vi "Raise Required Override Error.vi"(0 "RFFE Command in":refnum<class "RFFE Command.lvclass">, 5 "VI Refnum in (This VI)":refnum<vi>, 11 "error in (no error)":errorcluster) -> (4 "RFFE Command out":refnum<class "RFFE Command.lvclass">, 6 "VI Refnum out":refnum<vi>, 15 "error out":errorcluster)   [LabVIEW 2018, in "MIPI RFFE API.lvlib" / "RFFE Command.lvclass"]
uses:
  RFFE Command.lvclass
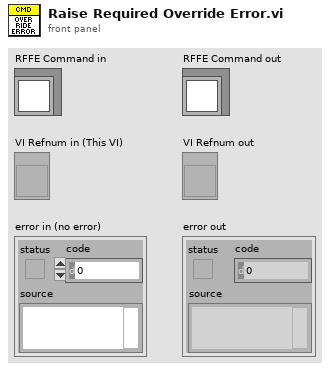
[diagram p1: front panel]
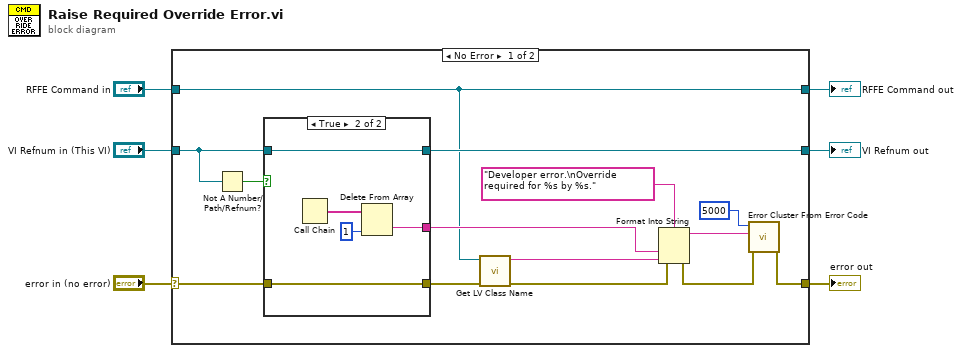
[diagram p0: block diagram]
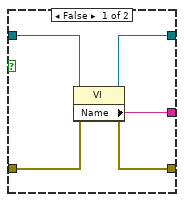
[diagram p2: hidden frame]
diagram:
  n1 = case shown="No Error" "error in (no error)" {
    selector: "error in (no error)" -> [w13 w33]
    tunnel: [w16 w33] -> w5
    tunnel: "VI Refnum in (This VI)" -> [w14 w32]
    tunnel: [w12 w32] -> w3
    tunnel: "RFFE Command in" -> [w7 w31]
    tunnel: [w7 w31] -> w1
    frame No Error {
      n2 = Not A Number/Path/Refnum?(number/path/refnum=w14) -> (NaN/Path/Refnum?=w15:bool)
      n3 = case shown="True" w15 {
        tunnel: w14 -> [w22 w30]
        tunnel: w13 -> [w25 w28]
        tunnel: [w21 w29] -> w11
        tunnel: [w24 w28] -> w10
        tunnel: [w23 w30] -> w12
        frame False {
          n4 = property class="VI"(reference=w22, error in=w25) -> (reference out=w23:refnum<vi>, error out=w24:errorcluster, "Name"=w21:string)
        }
        frame True {
          n5 = Call Chain() -> (call chain=w27:string[])
          n6 = Delete From Array(array=w27, index=1) -> (deleted portion=w29:string)  [unwired: 1 in, 1 out]
        }
      }
      n7 = call <vilib>:"Get LV Class Name.vi"("error in (no error)"=w10, "object"=w7) -> ("error out"=w9:errorcluster, "class name"=w8:string)  [unwired: 8 in]
      n8 = Format Into String(format string="Developer error.\nOverride required for %s by %s.", error in=w9, w11, w8) -> (resulting string=w18:string, error out=w17:errorcluster)  [unwired: 1 in]
      n9 = call <vilib>:"Error Cluster From Error Code.vi"("error in (no error)"=w17, "error message (\"\")"=w18, "error code (0)"=5000) -> ("error out"=w16:errorcluster)  [unwired: 6 in]
    }
    frame Error {
    }
  }
  "error out" <- w5
  "VI Refnum out" <- w3
  "RFFE Command out" <- w1
